vi "Set Body (JSON).vi"(8 "error in (no error)":errorcluster, 10 "Body (as JSON)":string, 11 "Response in":refnum<class "Response.lvclass">) -> (0 "error out":errorcluster, 3 "Response out":refnum<class "Response.lvclass">)   [LabVIEW 2023, in "Response.lvclass"]
uses:
  Response.lvclass
  Response.lvclass/Response.ctl
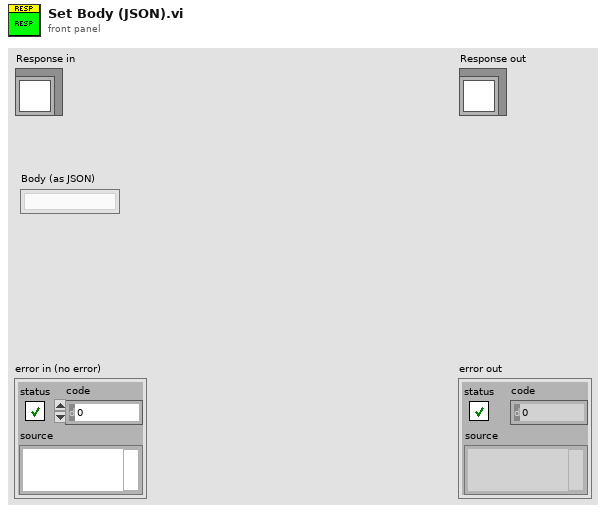
[diagram p1: front panel]
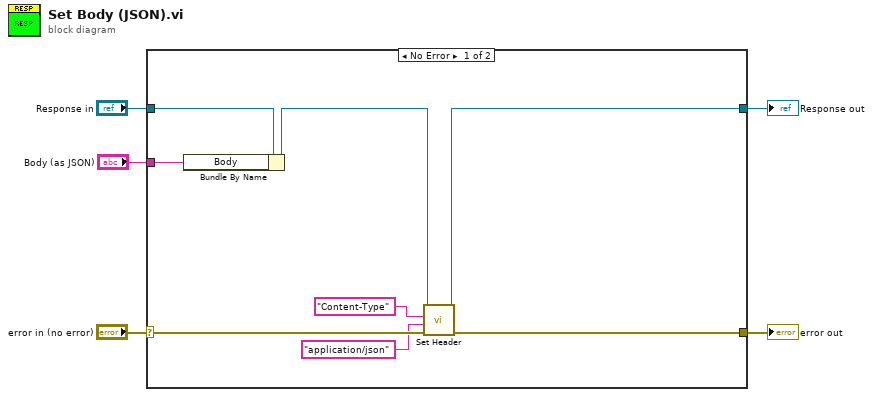
[diagram p0: block diagram]
diagram:
  n1 = case shown="No Error" "error in (no error)" {
    selector: "error in (no error)" -> [w11 w15]
    tunnel: [w10 w15] -> w4
    tunnel: [w8 w14] -> w2
    tunnel: "Response in" -> [w13 w14]
    tunnel: "Body (as JSON)" -> [w12 _]
    frame No Error {
      n2 = Bundle By Name(cluster=w13, "Body"=w12) -> (w9:refnum<class "Response.lvclass">)
      n3 = call "Set Header.vi"("error in (no error)"=w11, "Value"="application/json" ("Delimiter"), "Header"="Content-Type" ("Delimiter"), "Response in"=w9) -> ("error out"=w10:errorcluster, "Response out"=w8:refnum<class "Response.lvclass">)  [unwired: 5 in, 1 out]
    }
    frame Error {
    }
  }
  "error out" <- w4
  "Response out" <- w2
